vi "Correct_RD_Files.vi"() -> ()   [LabVIEW 2010]
panel:
  out "error out":errorcluster
  out "Number of strings found":i32
  out "Current File Number":i32
  out "No of Files Changed":i32
  out "Current FIlename":path
  in  "stop":bool
  out "Total Number of Files":i32
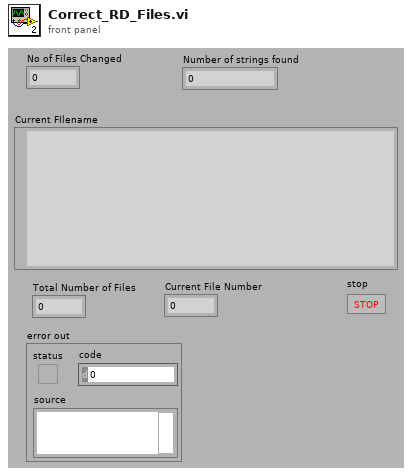
[diagram p1: front panel]
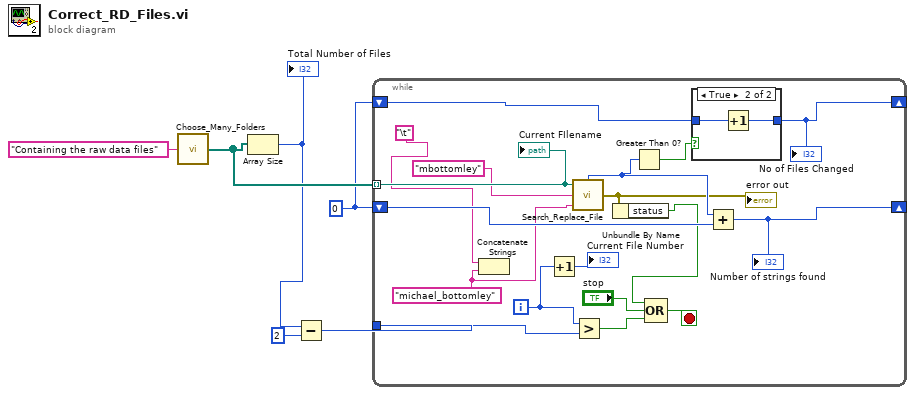
[diagram p0: block diagram]
diagram:
  w2 = 0
  n1 = call "Choose_Many_Folders.vi"("Purpose of choosing folder"="Containing the raw data files") -> ("Files"=w6:path[])
  n2 = Array Size(array=w6) -> (size(s)=w4:i32)
  "Total Number of Files" <- w4
  n3 = Subtract(x=w4, y=2) -> (x-y=w5:i32)
  n4 = while {
    tunnel: w6 -> [w24] mode=indexing
    tunnel: w5 -> [w23]
    shift-right: [w19] -> _
    shift-left: w2 -> [w18]
    shift-right: [w14] -> _
    shift-left: w2 -> [w15]
    i -> [w13]
    stop <- w20 stop-if-true
    w7 = "michael_bottomley" ("Replace_String")
    n5 = Concatenate Strings("\t", w7) -> ()  [unwired: 1 out]
    n6 = Increment(x=w13) -> (x+1=→"Current File Number":i32)
    n7 = call "Search_Replace_File.vi"("Replace_String"=w7, "Search_String"="mbottomley", "Path"=w24) -> ("error out"=w11:errorcluster, "Number Found"=w17:i32)
    "error out" <- w11
    n8 = Greater?(x=w13, y=w23) -> (0:w22:bool)
    n9 = Unbundle By Name(w11) -> ("status"=w10:bool)
    n10 = Greater Than 0?(x=w17) -> (x > 0?=w16:bool)
    n11 = Compound Arithmetic op=OR(w10, "stop", w22) -> (w20:bool)
    n12 = case shown="True" w16 {
      tunnel: w15 -> [w25 w27]
      tunnel: [w25 w26] -> w14
      frame False {
      }
      frame True {
        n13 = Increment(x=w27) -> (x+1=w26:i32)
      }
    }
    "No of Files Changed" <- w14
    n14 = Add(x=w17, y=w18) -> (x+y=w19:i32)
    "Number of strings found" <- w19
    "Current FIlename" <- w24
  }
